vi "WBRT Manual Control.vi"(0 "WBRT State In":T1 {"Trajectory Data" format="%0.3f"; "Filter Data"."Stop Frequency (Equi-Ripple)" format="%0.3f"; "Filter Data"."Pass Frequency" format="%0.3f"}, 2 "Manual Motor Control":bool, 4 "Lock together":bool=TRUE, 5 "error in (no error)":errorcluster, 6 "Right Motor (0-100%)":dbl, 7 "Stop In":bool, 8 "Left Motor (0-100%)":dbl=20.0, 9 "Landing Factor":dbl=0.1) -> (10 "Left Motor Display":dbl=-1.4210854715202004e-14, 12 "Right Motor Display":dbl=-1.4210854715202004e-14, 13 "Stop Out":bool, 14 "WBRT State Out":T1 {"Trajectory Data" format="%0.3f"; "Filter Data"."Stop Frequency (Equi-Ripple)" format="%0.3f"; "Filter Data"."Pass Frequency" format="%0.3f"}, 19 "error out":errorcluster)   [LabVIEW 2012]
uses:
  Custom Controls/WBRT State.ctl
  Custom Controls/WBRT Encoders.ctl
  Custom Controls/WBRT SPI Data.ctl
  Custom Controls/WBRT Filter Data.ctl
  Custom Controls/WBRT Filter Type.ctl
  FPGA Samples/spi_single port_example/Host API/Controls/FPGA SPI_FPGA Ref.ctl
  Custom Controls/WBRT Setpoints.ctl
  Custom Controls/WBRT Commands.ctl
  Custom Controls/WBRT Gains.ctl
  Custom Controls/WBRT Global Variables.ctl
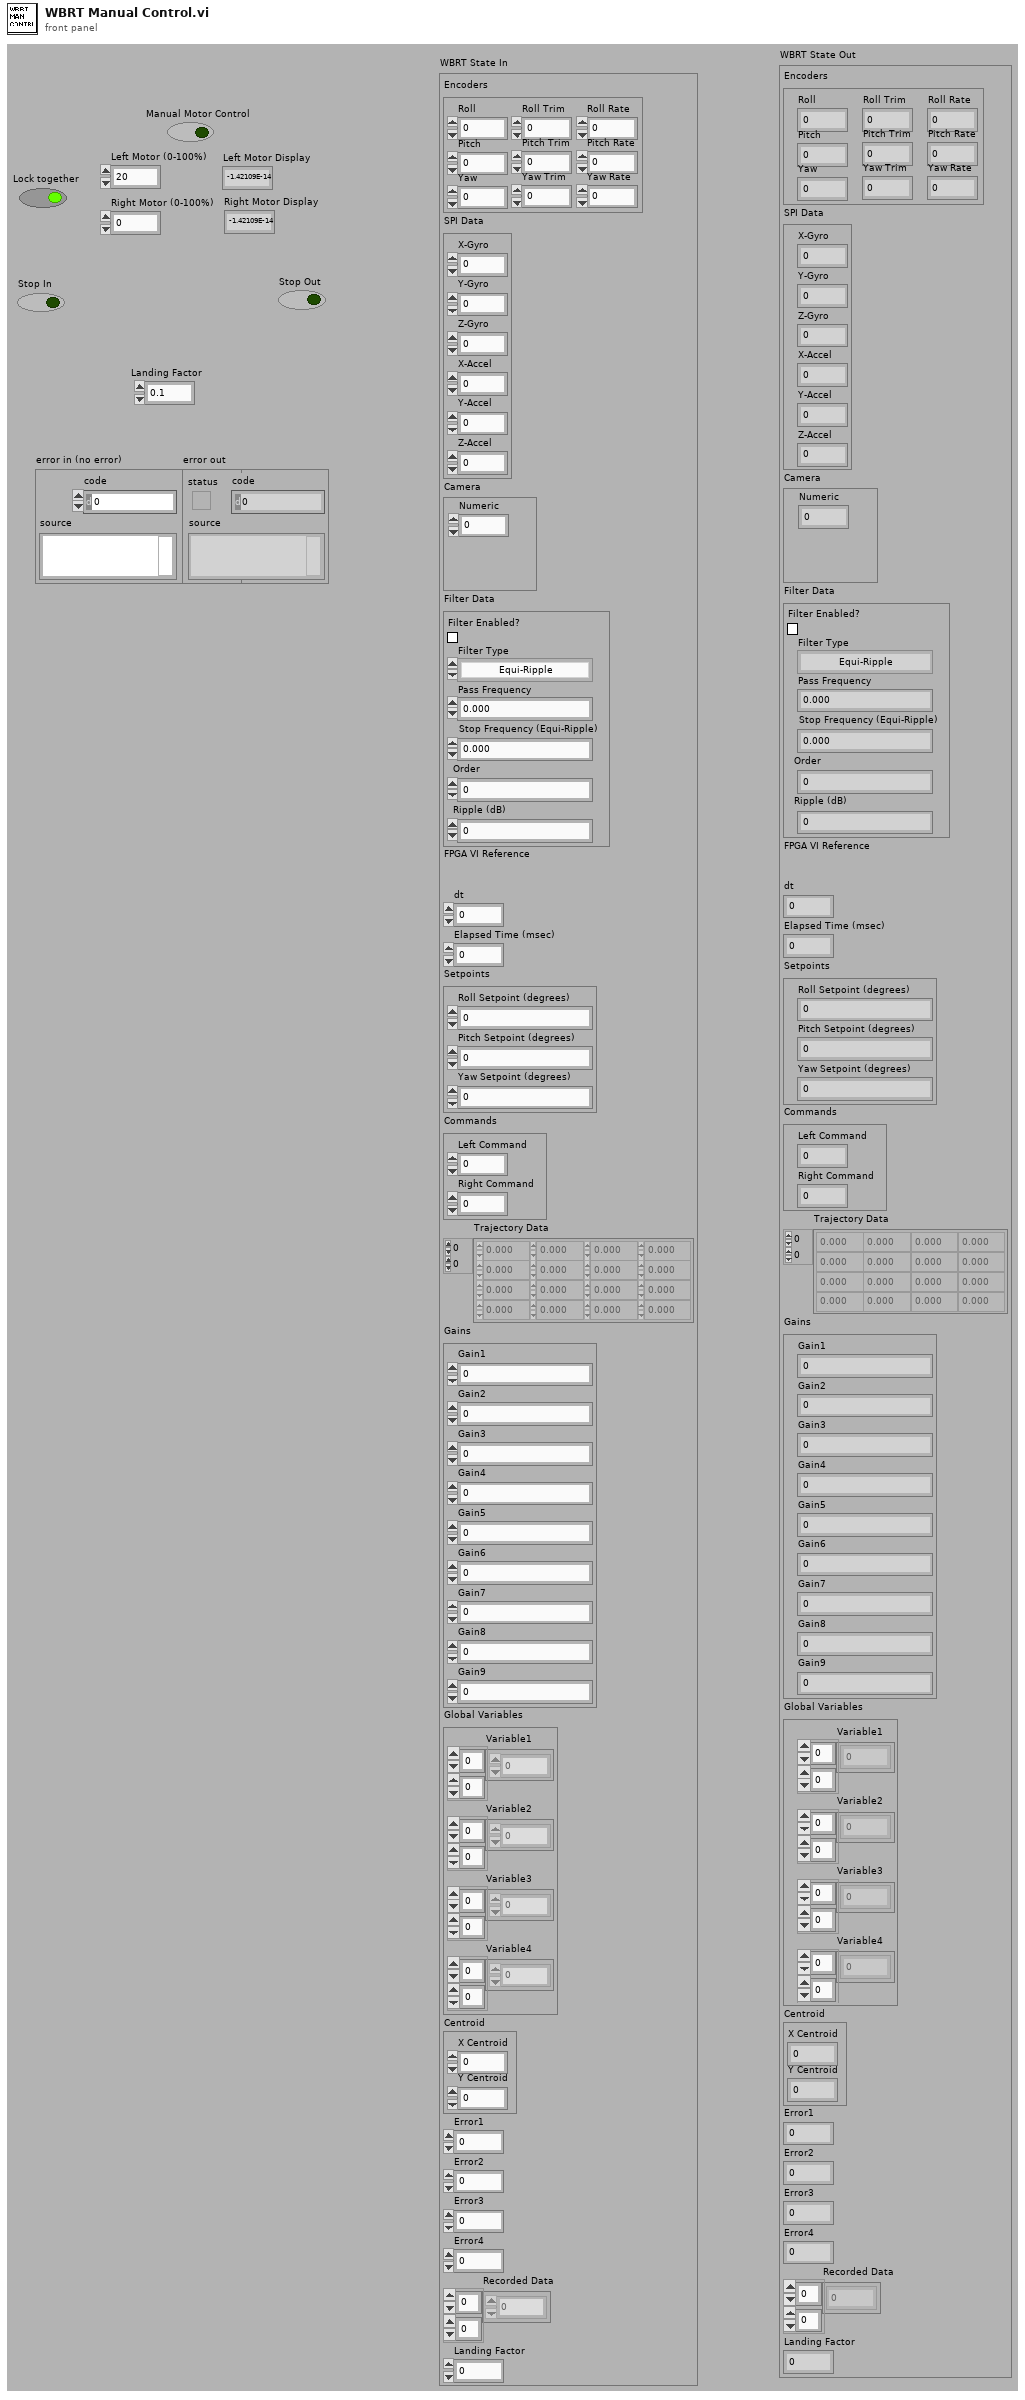
[diagram p1: front panel]
types:
  T1 = typedef "WBRT State.ctl" = cluster{"Encoders":T2, "SPI Data":T3, "Camera":cluster{"Numeric":dbl}, "Filter Data":T4, "FPGA VI Reference":T6, "dt":dbl, "Elapsed Time (msec)":u32, "Setpoints":T7, "Commands":T8, "Trajectory Data":dbl[][], "Gains":T9, "Global Variables":T10, "Centroid":cluster{"X Centroid":sgl, "Y Centroid":sgl}, "Error1":dbl, "Error2":dbl, "Error3":dbl, "Error4":dbl, "Recorded Data":dbl[][], "Landing Factor":dbl}
  T2 = typedef "WBRT Encoders.ctl" = cluster{"Roll":dbl, "Pitch":dbl, "Yaw":dbl, "Roll Trim":dbl, "Pitch Trim":dbl, "Yaw Trim":dbl, "Roll Rate":dbl, "Pitch Rate":dbl, "Yaw Rate":dbl}
  T3 = typedef "WBRT SPI Data.ctl" = cluster{"X-Gyro":dbl, "Y-Gyro":dbl, "Z-Gyro":dbl, "X-Accel":dbl, "Y-Accel":dbl, "Z-Accel":dbl}
  T4 = typedef "WBRT Filter Data.ctl" = cluster{"Filter Enabled?":bool, "Filter Type":T5, "Pass Frequency":dbl, "Stop Frequency (Equi-Ripple)":dbl, "Order":i32, "Ripple (dB)":dbl}
  T5 = typedef "WBRT Filter Type.ctl" = enum16{"Equi-Ripple", "Butterworth", "Chebyshev"}
  T6 = typedef "FPGA SPI_FPGA Ref.ctl" = refnum<k20>
  T7 = typedef "WBRT Setpoints.ctl" = cluster{"Roll Setpoint (degrees)":dbl, "Pitch Setpoint (degrees)":dbl, "Yaw Setpoint (degrees)":dbl}
  T8 = typedef "WBRT Commands.ctl" = cluster{"Left Command":dbl, "Right Command":dbl}
  T9 = typedef "WBRT Gains.ctl" = cluster{"Gain1":dbl, "Gain2":dbl, "Gain3":dbl, "Gain4":dbl, "Gain5":dbl, "Gain6":dbl, "Gain7":dbl, "Gain8":dbl, "Gain9":dbl}
  T10 = typedef "WBRT Global Variables.ctl" = cluster{"Variable1":dbl[][], "Variable2":dbl[][], "Variable3":dbl[][], "Variable4":dbl[][]}
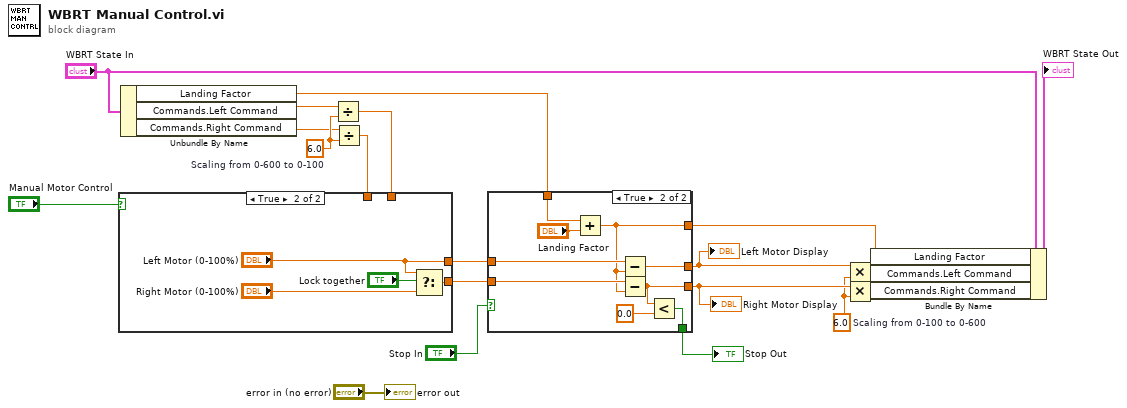
[diagram p0: block diagram]
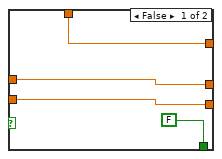
[diagram p2: hidden frame]
diagram:
  w14 = 6.0  # Scaling from 0-100 to 0-600
  w7 = 6.0  # Scaling from 0-600 to 0-100
  n1 = Unbundle By Name("WBRT State In") -> ("Landing Factor"=w3:dbl, "Commands.Left Command"=w5:dbl, "Commands.Right Command"=w4:dbl)
  n2 = Divide(x=w5, y=w7) -> (x/y=w10:dbl)
  n3 = Divide(x=w4, y=w7) -> (x/y=w11:dbl)
  n4 = case shown="True" "Manual Motor Control" {
    tunnel: [w21 w26] -> w17
    tunnel: [w22 "Left Motor (0-100%)"] -> w15
    tunnel: w10 -> [w22 _]
    tunnel: w11 -> [w21 _]
    frame False {
    }
    frame True {
      n5 = Select(t="Left Motor (0-100%)", s="Lock together", f="Right Motor (0-100%)") -> (s? t:f=w26:dbl)
    }
  }
  n6 = case shown="True" "Stop In" {
    tunnel: w15 -> [w30 w37]
    tunnel: [w30 w34] -> w16
    tunnel: w17 -> [w29 w36]
    tunnel: [w29 w32] -> w18
    tunnel: [w27 w35] -> w2
    tunnel: w3 -> [w27 w38]
    tunnel: [FALSE w33] -> w20
    frame False {
    }
    frame True {
      n7 = Add(x=w38, y="Landing Factor") -> (x+y=w35:dbl)
      n8 = Subtract(x=w37, y=w35) -> (x-y=w34:dbl)
      n9 = Subtract(x=w36, y=w35) -> (x-y=w32:dbl)
      n10 = Less?(x=w32, y=0.0) -> (x < y?=w33:bool)
    }
  }
  "Left Motor Display" <- w16
  "Right Motor Display" <- w18
  "Stop Out" <- w20
  n11 = Multiply(x=w16, y=w14) -> (x*y=w12:dbl)
  n12 = Multiply(x=w18, y=w14) -> (x*y=w13:dbl)
  n13 = Bundle By Name(cluster="WBRT State In", "Landing Factor"=w2, "Commands.Left Command"=w12, "Commands.Right Command"=w13) -> (→"WBRT State Out":T1)
  "error out" <- "error in (no error)"
